vi "RT2.vi"() -> ()   [LabVIEW 2013]
uses:
  <vilib>/FPGAPlugInAG/cRIO-9076/niLvFpga_Open_cRIO-9076.vi
  <vilib>/rvi/interface/common/dynamic/niFpgaDynamicAddResources.vi
  <vilib>/rvi/interface/common/niFpgaWaitOnOcc.vi
  <vilib>/Utility/error.llb/Error Cluster From Error Code.vi
  <vilib>/rvi/errors/niLvFpgaAdjustHostInterfaceError.vi
  <vilib>/FPGAPlugInAG/Dynamic/niLvFpga_Close_Dynamic.vi
  <vilib>/rvi/interface/nirviOpenFPGA/nirviOpenFPGA.xnode
  FPGA Bitfiles/PRL040515-withRL_FPGATarget_FPGA_chxCmvBjSj8.lvbitx
  FPGA.vi
  <vilib>/rvi/interface/nirviReadWriteControl/nirviReadWriteControl.xnode
  <vilib>/rvi/interface/nirviCloseFPGA/nirviCloseFPGA.xnode
  <vilib>/rvi/interface/Simulation/niFpgaSimulationCallBeginRW.vi
  NiFpgaLv.dll
panel:
  in  "stop":bool
  out "output cluster 2":T1
  in  "Hold Time":sgl=5000.0
  out "Loop period monitoring 2":u8
  in  "FPGA Loop  Timer":u8=100
  in  "Input pick":u16
  in  "alpha":sgl=1.81246
  in  "Frequency of oscillation":sgl=0.64
  in  "Scaling":sgl=120.0
  out "Loop period from PMU":u32
  out "Loop period monitoring":u32
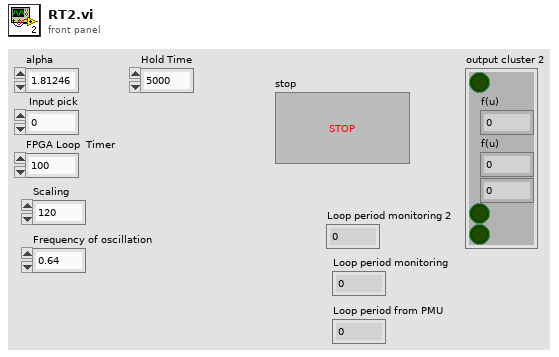
[diagram p1: front panel]
types:
  T1 = cluster{bool, "f(u)":sgl, "f(u)":sgl, sgl, bool, bool}
  T2 = cluster{"Parameters":cluster{"Ts":sgl, "kappaav":sgl, "kappaph":sgl, "mu":sgl}}
  T3 = cluster{"Voltage":sgl, "Current":sgl, "Power":sgl, "Load Change":sgl}
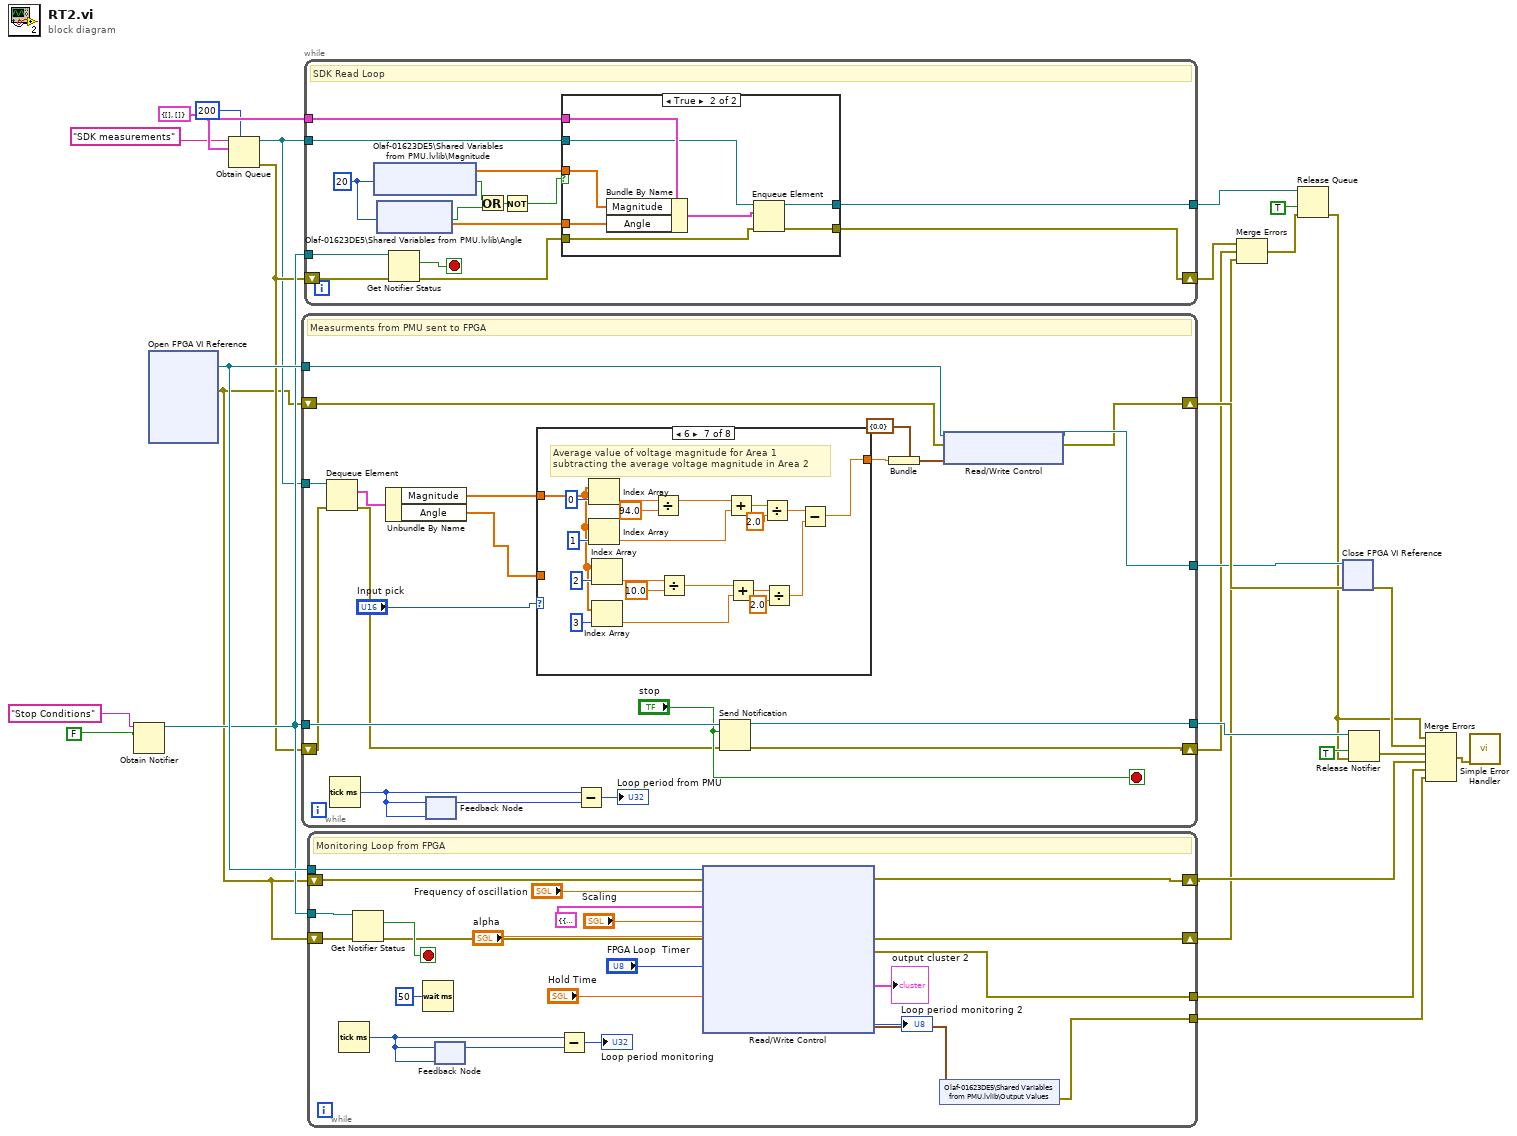
[diagram p0: block diagram]
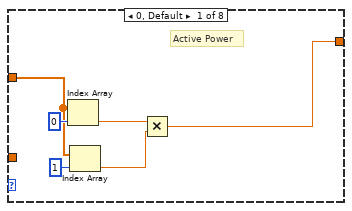
[diagram p3: hidden frame]
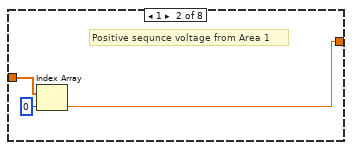
[diagram p4: hidden frame]
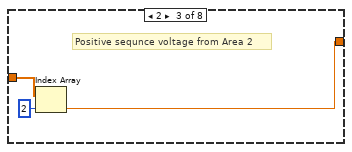
[diagram p5: hidden frame]
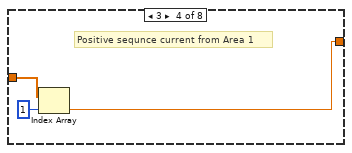
[diagram p6: hidden frame]
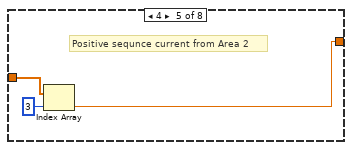
[diagram p7: hidden frame]
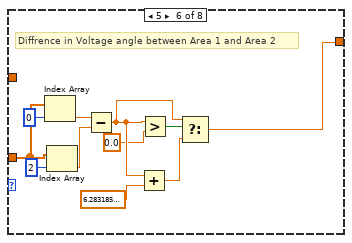
[diagram p8: hidden frame]
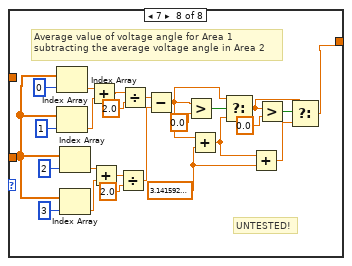
[diagram p9: hidden frame]
diagram:
  w16 = cluster{"Magnitude":sgl[], "Angle":sgl[]} {"Magnitude"=[], "Angle"=[]} ("input cluster")
  n1 = Obtain Notifier(name (unnamed)="Stop Conditions", notification data type=FALSE ("stop")) -> (notifier out=w8:refnum<notifier>)  [unwired: 2 in, 2 out]
  n2 = xnode "Open FPGA VI Reference"() -> ("FPGA VI Reference Out"=w26:refnum<k20>, "error out"=w5:errorcluster)  [unwired: 2 in]
  n3 = Obtain Queue(max queue size (-1, unlimited)=200, name (unnamed)="SDK measurements", element data type=w16) -> (queue out=w6:refnum<queue>, error out=w7:errorcluster)  [unwired: 2 in, 1 out]
  n4 = while {
    tunnel: w26 -> [w44]
    tunnel: [w48] -> w25
    tunnel: w8 -> [w41]
    tunnel: [w40] -> w18
    tunnel: w6 -> [w33]
    shift-right: [w29] -> w3
    shift-left: w7 -> [w32]
    shift-right: [w42] -> w27
    shift-left: w5 -> [w28]
    stop <- "stop" stop-if-true
    # "Measurments from PMU sent to FPGA"
    n5 = Dequeue Element(queue=w33, error in (no error)=w32) -> (element=w39:cluster{"Magnitude":sgl[], "Angle":sgl[]}, error out=w30:errorcluster)  [unwired: 1 in, 2 out]
    n6 = Tick Count (ms)() -> (millisecond timer value=w46:u32)
    n7 = Unbundle By Name(w39) -> ("Magnitude"=w34:sgl[], "Angle"=w35:sgl[])
    n8 = feedback #1(w46) -> (w45:u32)
    n9 = feedback-in #1(w46) -> ()
    n10 = case shown="6" "Input pick" {
      tunnel: w35 -> [_ _ _ _ _ w77 _ w108]
      tunnel: [w52 w55 w58 w61 w64 w67 w87 w98] -> w36
      tunnel: w34 -> [w51 w56 w59 w62 w65 _ w82 _]
      frame 0, Default {
        # "Active Power"
        n11 = Index Array(array=w51, index=0) -> (element=w50:sgl)
        n12 = Index Array(array=w51, index=1) -> (element=w49:sgl)
        n13 = Multiply(x=w50, y=w49) -> (x*y=w52:sgl)
      }
      frame 1 {
        # "Positive sequnce voltage from Area 1"
        n14 = Index Array(array=w56, index=0) -> (element=w55:sgl)
      }
      frame 2 {
        # "Positive sequnce voltage from Area 2"
        n15 = Index Array(array=w59, index=2) -> (element=w58:sgl)
      }
      frame 3 {
        # "Positive sequnce current from Area 1"
        n16 = Index Array(array=w62, index=1) -> (element=w61:sgl)
      }
      frame 4 {
        # "Positive sequnce current from Area 2"
        n17 = Index Array(array=w65, index=3) -> (element=w64:sgl)
      }
      frame 5 {
        # "Diffrence in Voltage angle between Area 1 and Area 2"
        n18 = Index Array(array=w77, index=0) -> (element=w74:sgl)
        n19 = Index Array(array=w77, index=2) -> (element=w73:sgl)
        n20 = Subtract(x=w74, y=w73) -> (x-y=w71:sgl)
        n21 = Add(x=w71, y=sgl 6.2831855) -> (x+y=w70:sgl)
        n22 = Greater?(x=w71, y=sgl 0.0 ("x")) -> (0:w72:bool)
        n23 = Select(t=w71, s=w72, f=w70) -> (s? t:f=w67:sgl)
      }
      frame 6 {
        # "Average value of voltage magnitude for Area 1 \nsubtracting the average voltage magnitude in Area 2"
        n24 = Index Array(array=w82, index=0) -> (element=w80:sgl)
        n25 = Index Array(array=w82, index=1) -> (element=w81:sgl)
        n26 = Index Array(array=w82, index=2) -> (element=w79:sgl)
        n27 = Index Array(array=w82, index=3) -> (element=w78:sgl)
        n28 = Divide(x=w80, y=sgl 94.0) -> (x/y=w85:sgl)
        n29 = Divide(x=w79, y=sgl 10.0) -> (x/y=w83:sgl)
        n30 = Add(x=w85, y=w81) -> (x+y=w93:sgl)
        n31 = Add(x=w83, y=w78) -> (x+y=w92:sgl)
        n32 = Divide(x=w93, y=sgl 2.0) -> (x/y=w89:sgl)
        n33 = Divide(x=w92, y=sgl 2.0) -> (x/y=w88:sgl)
        n34 = Subtract(x=w89, y=w88) -> (x-y=w87:sgl)
      }
      frame 7 {
        w101 = sgl 3.1415927 ("y")
        # "UNTESTED!"
        # "Average value of voltage angle for Area 1 \nsubtracting the average voltage angle in Area 2"
        n35 = Index Array(array=w108, index=0) -> (element=w118:sgl)
        n36 = Index Array(array=w108, index=1) -> (element=w117:sgl)
        n37 = Index Array(array=w108, index=2) -> (element=w116:sgl)
        n38 = Index Array(array=w108, index=3) -> (element=w115:sgl)
        n39 = Add(x=w118, y=w117) -> (x+y=w114:sgl)
        n40 = Add(x=w116, y=w115) -> (x+y=w113:sgl)
        n41 = Divide(x=w113, y=sgl 2.0) -> (x/y=w109:sgl)
        n42 = Divide(x=w114, y=sgl 2.0) -> (x/y=w110:sgl)
        n43 = Subtract(x=w110, y=w109) -> (x-y=w105:sgl)
        n44 = Greater?(x=w105, y=sgl 0.0) -> (0:w106:bool)
        n45 = Add(x=w105, y=w101) -> (x+y=w102:sgl)
        n46 = Select(t=w105, s=w106, f=w102) -> (s? t:f=w99:sgl)
        n47 = Add(x=w102, y=w101) -> (x+y=w100:sgl)
        n48 = Greater?(x=w99, y=sgl 0.0) -> (0:w103:bool)
        n49 = Select(t=w99, s=w103, f=w100) -> (s? t:f=w98:sgl)
      }
    }
    n50 = Subtract(x=w46, y=w45) -> (x-y=→"Loop period from PMU":u32)
    n51 = Send Notification(notification="stop", notifier=w41, error in (no error)=w30) -> (notifier out=w40:refnum<notifier>, error out=w29:errorcluster)
    n52 = Bundle(cluster=cluster{sgl} {0.0}, w36) -> (w38:cluster{sgl})
    n53 = xnode "Read/Write Control"("FPGA VI Reference In"=w44, "error in"=w28, "PMU measurments"=w38) -> ("FPGA VI Reference Out"=w48:refnum<k20>, "error out"=w42:errorcluster)
  }
  n54 = while {
    tunnel: w16 -> [w131]
    tunnel: w6 -> [w130]
    shift-right: [w128] -> w4
    shift-left: w7 -> [w123]
    tunnel: w8 -> [w127]
    tunnel: [w125] -> w13
    stop <- w126 stop-if-true
    w137 = 20 ("ms timeout (0)")
    # "SDK Read Loop"
    n55 = shared-variable "Olaf-01623DE5\\Shared Variables from PMU.lvlib\\Magnitude"(w137) -> (w133:sgl[], w136:bool)  [unwired: 1 in, 1 out]
    n56 = shared-variable "Olaf-01623DE5\\Shared Variables from PMU.lvlib\\Angle"(w137) -> (w132:sgl[], w135:bool)  [unwired: 1 in, 1 out]
    n57 = Get Notifier Status(notifier=w127, error in (no error)=w123) -> (current notification=w126:bool, error out=w124:errorcluster)  [unwired: 3 out]
    n58 = Or(x=w136, y=w135) -> (x .or. y?=w134:bool)
    n59 = Not(x=w134) -> (.not. x?=w129:bool)
    n60 = case shown="True" w129 {
      tunnel: w133 -> [_ w147]
      tunnel: w132 -> [_ w146]
      tunnel: w131 -> [_ w144]
      tunnel: w130 -> [w138 w143]
      tunnel: w124 -> [w139 w142]
      tunnel: [w139 w141] -> w128
      tunnel: [w138 w140] -> w125
      frame False {
      }
      frame True {
        n61 = Bundle By Name(cluster=w144, "Magnitude"=w147, "Angle"=w146) -> (w145:cluster{"Magnitude":sgl[], "Angle":sgl[]})
        n62 = Enqueue Element(queue=w143, element=w145, error in (no error)=w142) -> (queue out=w140:refnum<queue>, error out=w141:errorcluster)  [unwired: 1 in, 1 out]
      }
    }
  }
  n63 = while {
    tunnel: w26 -> [w169]
    tunnel: [w158] -> w22
    tunnel: [w157] -> w21
    tunnel: w8 -> [w152]
    shift-right: [w149] -> w9
    shift-left: w5 -> [w168]
    shift-right: [w150] -> w2
    shift-left: w5 -> [w148]
    stop <- w151 stop-if-true
    # "Monitoring Loop from FPGA"
    n64 = Tick Count (ms)() -> (millisecond timer value=w166:u32)
    n65 = Get Notifier Status(notifier=w152, error in (no error)=w148) -> (current notification=w151:bool, error out=w150:errorcluster)  [unwired: 3 out]
    n66 = Wait (ms)(milliseconds to wait=u32 50) -> ()  [unwired: 1 out]
    n67 = feedback #2(w166) -> (w165:u32)
    n68 = feedback-in #2(w166) -> ()
    n69 = Subtract(x=w166, y=w165) -> (x-y=→"Loop period monitoring":u32)
    n70 = xnode "Read/Write Control"("FPGA VI Reference In"=w169, "error in"=w168, "Frequency of oscillation"="Frequency of oscillation", "Frequency Estimator Settings"=T2 {"Parameters"={"Ts"=5e-05, "kappaav"=0.625, "kappaph"=0.5762, "mu"=0.7086}}, "Scaling"="Scaling", "alpha"="alpha", "FPGA Loop  Timer"="FPGA Loop  Timer", "Hold Time"="Hold Time") -> ("error out"=w149:errorcluster, "FPGA Error Out"=w158:errorcluster, "output cluster 2"=→"output cluster 2":T1, "Loop period monitoring"=→"Loop period monitoring 2":u8, "output cluster"=w163:T3)  [unwired: 1 out]
    n71 = shared-variable "Olaf-01623DE5\\Shared Variables from PMU.lvlib\\Output Values"(w163) -> (error out=w157:errorcluster)  [unwired: 1 in]
  }
  n72 = Merge Errors(w4, w3, w2) -> (w1:errorcluster)
  n73 = Release Queue(queue=w13, force destroy? (F)=TRUE, error in (no error)=w1) -> (error out=w10:errorcluster)  [unwired: 2 out]
  n74 = xnode "Close FPGA VI Reference"("FPGA VI Reference In"=w25, "error in"=w27) -> ("error out"=w24:errorcluster)
  n75 = Release Notifier(notifier=w18, force destroy? (F)=TRUE, error in (no error)=w10) -> (error out=w17:errorcluster)  [unwired: 2 out]
  n76 = Merge Errors(w10, w24, w17, w9, w22, w21) -> (w23:errorcluster)
  n77 = call <vilib>:"Simple Error Handler.vi"("error in (no error)"=w23) -> ()  [unwired: 4 in, 5 out]
